vi "Quadratic Formula.vi"() -> ()   [LabVIEW 2015]
panel:
  out "XY Graph":cluster{i32, dbl}[](graph)
  out "Answer 2":dbl
  out "Answer 1":dbl
  in  "C":dbl
  in  "B":dbl
  in  "A":dbl
  # "Y = aX^2 + bX + c"
  # "Finds the values of X when Y = 0"
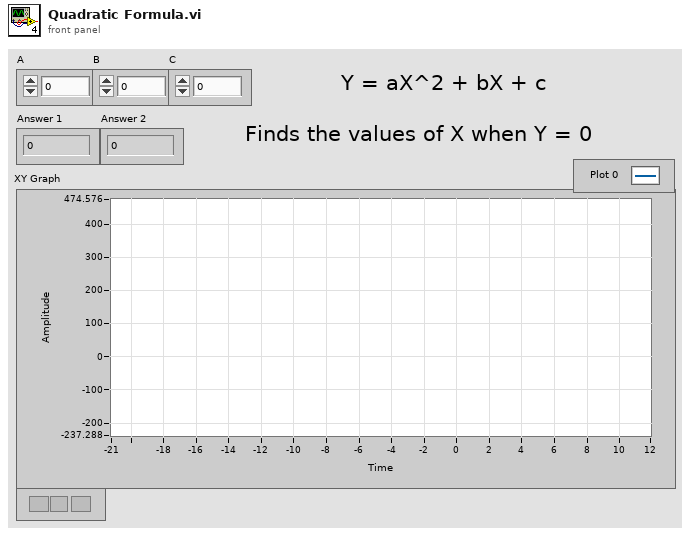
[diagram p1: front panel]
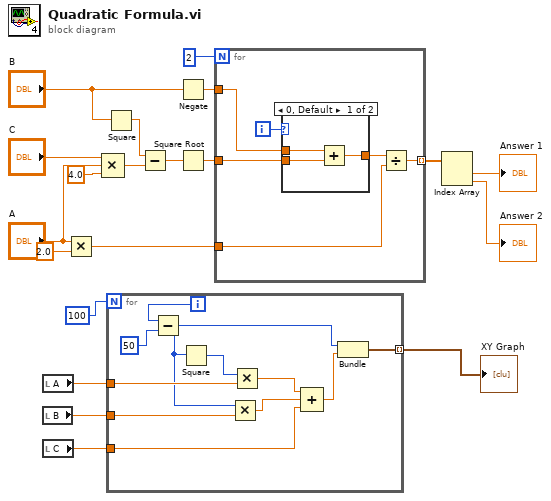
[diagram p0: block diagram]
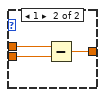
[diagram p2: hidden frame]
diagram:
  n1 = local read "A"() -> (w5:dbl)
  n2 = local read "B"() -> (w4:dbl)
  n3 = local read "C"() -> (w3:dbl)
  n4 = Multiply(x="A", y=2.0) -> (x*y=w11:dbl)
  n5 = Compound Arithmetic op=MULTIPLY("C", "A", 4.0 ("value")) -> (w15:dbl)
  n6 = Square(x="B") -> ()  [unwired: 1 out]
  n7 = for {
    N: 100 -> [_]
    tunnel: w5 -> [w27]
    tunnel: w4 -> [w26]
    tunnel: w3 -> [w23]
    tunnel: [w20] -> w2 mode=indexing
    i -> [w30]
    n8 = Subtract(x=w30, y=50) -> (x-y=w22:i32)
    n9 = Square(x=w22) -> (x^2=w28:i32)
    n10 = Multiply(x=w22, y=w26) -> (x*y=w24:dbl)
    n11 = Multiply(x=w28, y=w27) -> (x*y=w25:dbl)
    n12 = Compound Arithmetic op=ADD(w25, w24, w23) -> (w21:dbl)
    n13 = Bundle(w22, w21) -> (w20:cluster{i32, dbl})  [unwired: 1 in]
  }
  "XY Graph" <- w2
  n14 = Subtract(x="B", y=w15) -> (x-y=w14:dbl)
  n15 = Negate(x="B") -> (-x=w13:dbl)
  n16 = Square Root(x=w14) -> (sqrt(x)=w10:dbl)
  n17 = for {
    N: 2 -> [_]
    tunnel: w13 -> [w36]
    tunnel: w11 -> [w35]
    tunnel: w10 -> [w34]
    tunnel: [w31] -> w8 mode=indexing
    i -> [w32]
    n18 = case shown="0, Default" w32 {
      tunnel: w36 -> [w39 w42]
      tunnel: w34 -> [w38 w41]
      tunnel: [w37 w40] -> w33
      frame 0, Default {
        n19 = Add(x=w39, y=w38) -> (x+y=w37:dbl)
      }
      frame 1 {
        n20 = Subtract(x=w42, y=w41) -> (x-y=w40:dbl)
      }
    }
    n21 = Divide(x=w33, y=w35) -> (x/y=w31:dbl)
  }
  n22 = Index Array(array=w8) -> (element #1=→"Answer 1":dbl, element #2=→"Answer 2":dbl)  [unwired: 2 in]
